vi "robot - Point on Circle.vi"(6 "Scale Factor":dbl=1.0, 9 "Angle":dbl, 10 "Radius":dbl, 11 "Rect In":T2) -> (0 "Scaled Rect Out":T1, 1 "Rect Out":T1, 2 "scaled point":cluster{"x":dbl, "y":dbl}, 3 "point":cluster{"x":dbl, "y":dbl})   [LabVIEW 2023]
doc: "This VI returns the point at which a radius line at the given angle (in radians) meets the circle defined by center and radius."
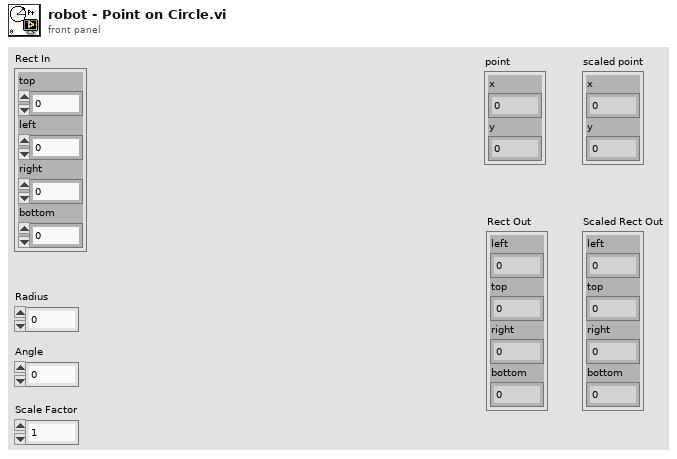
[diagram p1: front panel]
types:
  T1 = cluster{"left":dbl, "top":dbl, "right":dbl, "bottom":dbl}
  T2 = cluster{"top":dbl, "left":dbl, "right":dbl, "bottom":dbl}
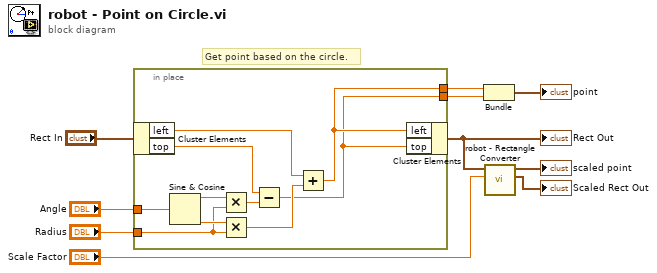
[diagram p0: block diagram]
diagram:
  # "Get point based on the circle."
  n1 = in-place {
    in-place-border: "Angle" -> [w20]
    in-place-border: "Radius" -> [w15]
    in-place-border: [w12] -> w8
    in-place-border: [w11] -> w7
    n2 = in-place-cluster #1("Rect In") -> ("left"=w14:dbl, "top"=w13:dbl)
    n3 = Sine & Cosine(0:w20) -> (1:w18:dbl, 2:w19:dbl)
    n4 = Multiply(x=w18, y=w15) -> (x*y=w17:dbl)
    n5 = Multiply(x=w19, y=w15) -> (x*y=w16:dbl)
    n6 = Subtract(x=w13, y=w17) -> (x-y=w11:dbl)
    n7 = Add(x=w14, y=w16) -> (x+y=w12:dbl)
    n8 = in-place-cluster #1("left"=w12, "top"=w11) -> (w1:T2)
  }
  "Rect Out" <- w1
  n9 = Bundle(w8, w7) -> (→"point":cluster{dbl, dbl})  [unwired: 1 in]
  n10 = call "robot - Rectangle Converter.vi"("Scale Factor"="Scale Factor", "Rect"=w1) -> ("Rect Out"=→"Scaled Rect Out":T1, "Center"=→"scaled point":cluster{"x":dbl, "y":dbl})  [unwired: 8 in]
